vi "Get Favorite Color.vi"(8 "error in":errorcluster, 11 "Zhenyu in":refnum<class "Zhenyu.lvclass">) -> (0 "error out":errorcluster, 2 "Favorite Color":u32(colorbox), 3 "Zhenyu out":refnum<class "Zhenyu.lvclass">)   [LabVIEW 2024, in "Zhenyu.lvclass"]
uses:
  Zhenyu.lvclass
  Zhenyu.lvclass/Zhenyu.ctl
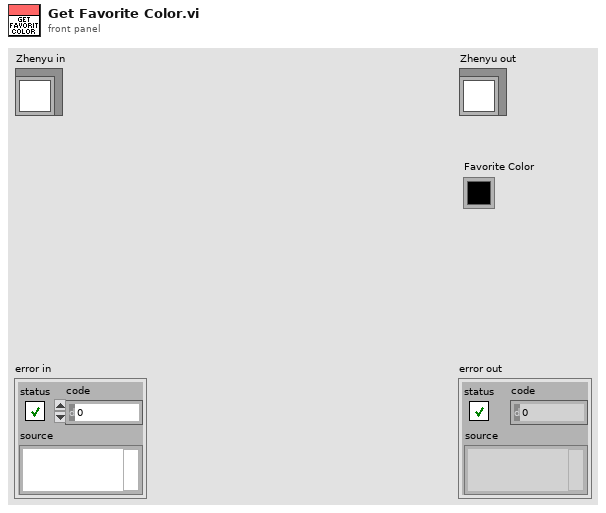
[diagram p1: front panel]
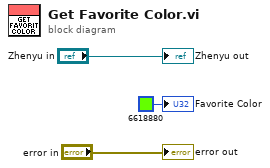
[diagram p0: block diagram]
diagram:
  "error out" <- "error in"
  "Zhenyu out" <- "Zhenyu in"
  "Favorite Color" <- u32 6618880 ("Favorite Color")
